vi "ReadPickeringConfig.vi"(8 "error in (no error)":errorcluster) -> (0 "error out":errorcluster, 2 "Pickering Config":T1)   [LabVIEW 2016, in "pickering.lvclass"]
uses:
  pickering.lvclass
  Typedefs/PickeringConfig-Cluster.ctl
  Typedefs/PickeringXConfig-Cluster.ctl
  Typedefs/PickeringYConfig-Cluster.ctl
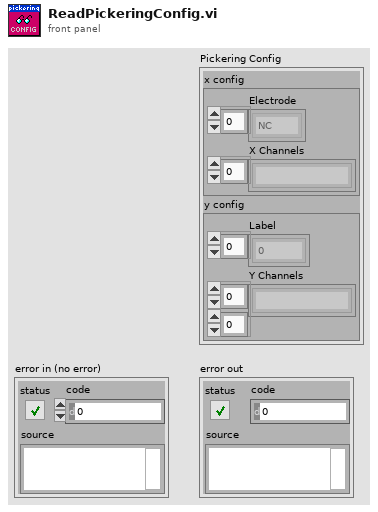
[diagram p1: front panel]
types:
  T1 = typedef "pickering.lvclass/PickeringConfig-Cluster.ctl" = cluster{"x config":T2, "y config":T3}
  T2 = typedef "pickering.lvclass/PickeringXConfig-Cluster.ctl" = cluster{"Electrode":enum16{"NC", "26", "27", "28", "1", "2", "3", "4", "5", "6", "7", "8", "9", "10", "11", "12", "13", "14", "15", "16", "17", "18", "19", "20", "21", "22", "23", "24", "25"}[], "X Channels":string[]}
  T3 = typedef "pickering.lvclass/PickeringYConfig-Cluster.ctl" = cluster{"Label":u16[], "Y Channels":string[][]}
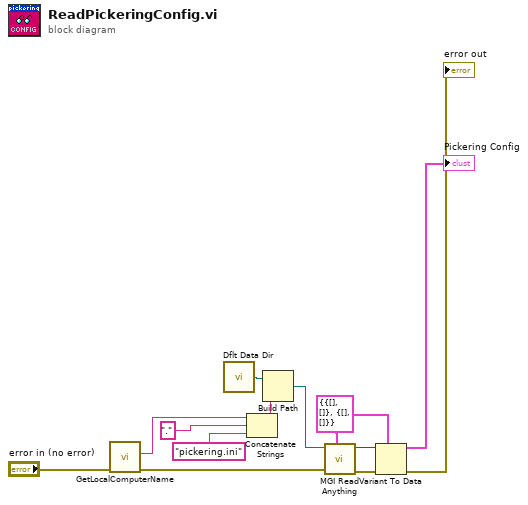
[diagram p0: block diagram]
diagram:
  w4 = T1 {"x config"={"Electrode"=[], "X Channels"=[]}, "y config"={"Label"=[], "Y Channels"=[]}} ("cluster")
  n1 = call <userlib>:"GetLocalComputerName.vi"("error in (no error)"="error in (no error)") -> ("error out"=w12:errorcluster, "Name"=w11:string)  [unwired: 8 in, 1 out]
  n2 = call <vilib>:"Dflt Data Dir.vi"() -> ("App:Default Data Directory"=w1:path)
  n3 = Concatenate Strings(w11, "." ("string"), "pickering.ini" ("name or relative path")) -> (w8:string)
  n4 = Build Path(base path=w1, name or relative path=w8) -> (appended path=w13:path)
  n5 = call <userlib>:"MGI Read Anything.vi"("Type of Anything"=w4, "Error In"=w12, "Path (dialog)"=w13) -> ("Error Out"=w2:errorcluster, "Anything"=w3:variant)  [unwired: 5 in, 2 out]
  n6 = Variant To Data(error in=w2, type=w4, Variant=w3) -> (data=→"Pickering Config":T1, error out=→"error out":errorcluster)
